vi "Write.vi"(7 "Map id":i32, 8 "Error In":errorcluster, 10 "Data":dbl[](array[numeric]), 11 "Indices":i32[](array[numeric])) -> (0 "Error Out":errorcluster)   [LabVIEW 2018]
uses:
  SharedMemoryTest.dll
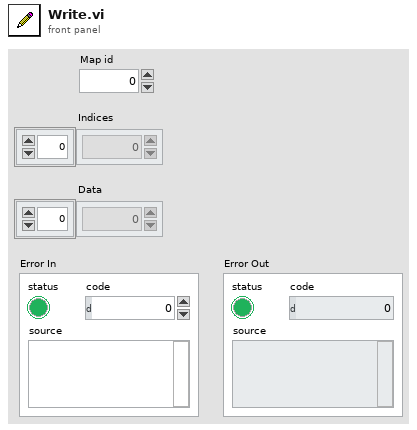
[diagram p1: front panel]
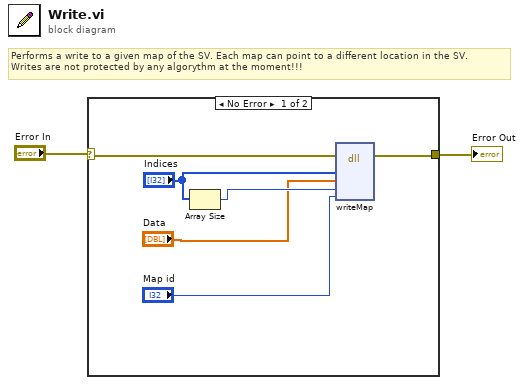
[diagram p0: block diagram]
diagram:
  # "Performs a write to a given map of the SV. Each map can point to a different location in the SV.\nWrites are not protected by any algorythm at the moment!!!"
  n1 = case shown="No Error" "Error In" {
    selector: "Error In" -> [w8 w9]
    tunnel: [w7 w9] -> w1
    frame No Error {
      n2 = Array Size(array="Indices") -> (size(s)=w5:i32)
      n3 = dll-call lib="C:/Users/jaros/Desktop/UIF_StateVector/SV operations/SharedMemoryTest.dll" fn="writeMap"(error in=w8, "idx"="Indices", "data"="Data", "length"=w5, "map id"="Map id") -> (error out=w7:errorcluster)  [unwired: 7 in, 1 out]
    }
    frame Error {
    }
  }
  "Error Out" <- w1
